vi "Keithley 6517A Display Read.vi"(0 "GPIB address":string="27", 1 "error in":T1) -> (2 "primary display":string, 3 "secondary display":string, 4 "error out":T1)   [LabVIEW 2024]
doc: "This VI is used to read the primary and secondary display of the instrument as an ASCII text string."
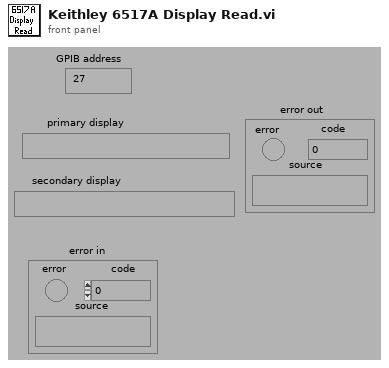
[diagram p1: front panel]
types:
  T1 = cluster{"error":bool, "code":i32, "source":string}
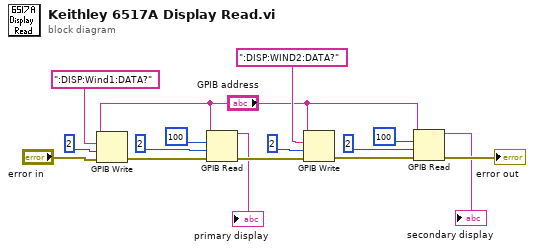
[diagram p0: block diagram]
diagram:
  n1 = GPIB Write(0:"GPIB address", 1:":DISP:Wind1:DATA?", 2:2, 3:"error in") -> (6:w12:errorcluster)  [unwired: 1 in, 1 out]
  n2 = GPIB Read(0:"GPIB address", 1:100, 2:2, 3:w12) -> (5:→"primary display":string, 7:w13:errorcluster)  [unwired: 1 in, 1 out]
  n3 = GPIB Write(0:"GPIB address", 1:":DISP:WIND2:DATA?", 2:2, 3:w13) -> (6:w14:errorcluster)  [unwired: 1 in, 1 out]
  n4 = GPIB Read(0:"GPIB address", 1:100, 2:2, 3:w14) -> (5:→"secondary display":string, 7:→"error out":errorcluster)  [unwired: 1 in, 1 out]
